vi "store_nodes.vi"(0 "destination_vectorstore in":refnum<class "destination_vectorstore.lvclass">, 5 "nodes":refnum<class "data_node.lvclass">[](array[class]), 11 "error in (no error)":errorcluster) -> (4 "destination_vectorstore out":refnum<class "destination_vectorstore.lvclass">, 15 "error out":errorcluster)   [LabVIEW 2020, in "destination_vectorstore.lvclass"]
uses:
  destination_vectorstore.lvclass
  data/data_node/data_node.lvclass
  destination_vectorstore.lvclass/destination_vectorstore.ctl
  vectorstore/abstract_vector_base/vector.ctl
  vectorstore/abstract_vector_base/abstract_vector_base.lvclass
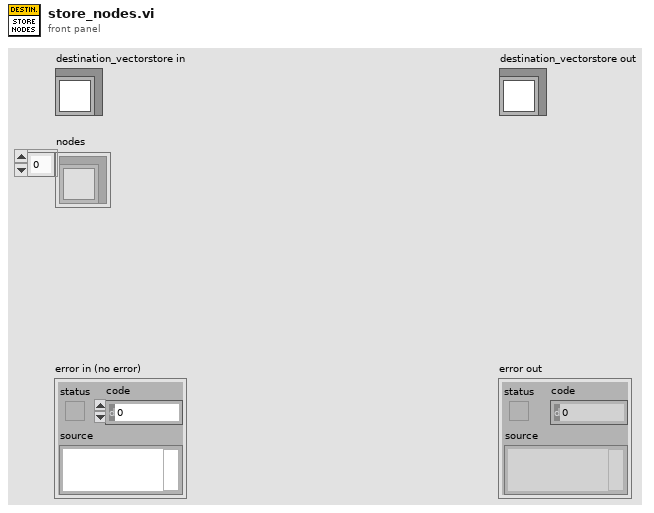
[diagram p1: front panel]
types:
  T1 = typedef "abstract_vector_base.lvclass/vector.ctl" = cluster{"id":string, "vector":dbl[], "text":string, "metadata":cluster{"key":string, "value":string}[]}
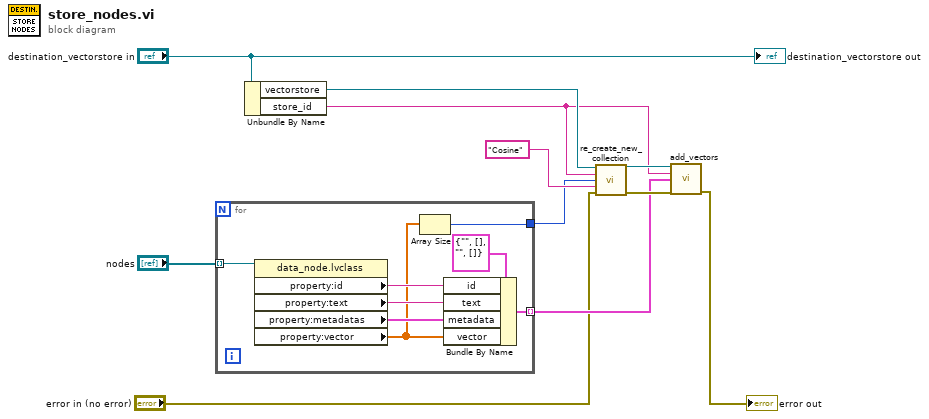
[diagram p0: block diagram]
diagram:
  n1 = for {
    tunnel: "nodes" -> [w19] mode=indexing
    tunnel: [w14] -> w6 mode=indexing
    tunnel: [w12] -> w1
    n2 = property class="data_node.lvclass"(reference=w19) -> ("property:id"=w17:string, "property:text"=w16:string, "property:metadatas"=w15:cluster{"key":string, "value":string}[], "property:vector"=w13:dbl[])  [unwired: 1 in, 2 out]
    n3 = Array Size(array=w13) -> (size(s)=w12:i32)
    n4 = Bundle By Name(cluster=T1 {"id"="", "vector"=[], "text"="", "metadata"=[]} ("vector"), "id"=w17, "text"=w16, "metadata"=w15, "vector"=w13) -> (w14:T1)
  }
  n5 = Unbundle By Name("destination_vectorstore in") -> ("vectorstore"=w9:refnum<class "abstract_vector_base.lvclass">, "store_id"=w8:string)
  n6 = call-dynamic "re_create_new_collection.vi"("abstract_vector_base in"=w9, "collection_name"=w8, "vector_size"=w1, "distance"="Cosine", "error in (no error)"="error in (no error)") -> ("abstract_vector_base out"=w11:refnum<class "abstract_vector_base.lvclass">, "error out"=w10:errorcluster)  [unwired: 9 in]
  n7 = call-dynamic "add_vectors.vi"("abstract_vector_base in"=w11, "colection_name"=w8, "vectors"=w6, "error in (no error)"=w10) -> ("error out"=→"error out":errorcluster)  [unwired: 10 in, 1 out]
  "destination_vectorstore out" <- "destination_vectorstore in"
